vi "Draw Target Vr2.vi"(1 "Color":u32(colorbox)=16448250, 2 "Thickness":i32=3, 3 "Original Image":T1(plugin-control)) -> (0 "Image Out":T1(plugin-control))   [LabVIEW 2012]
uses:
  <resource>/objmgr/IMAQImage.rc
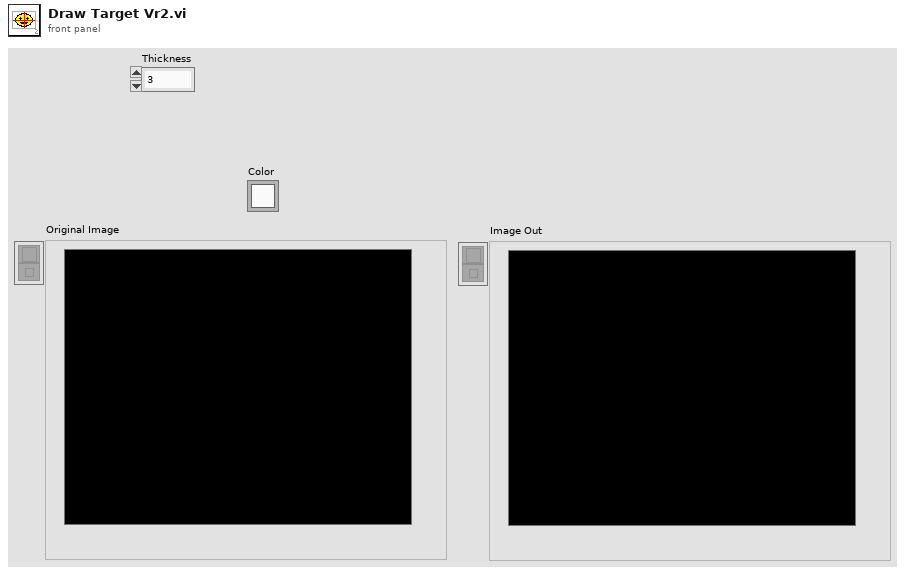
[diagram p1: front panel]
types:
  T1 = typedef "IMAQ Image.ctl" = refnum<image>
  T2 = cluster{"Left":i32, "Top":i32, "Right":i32, "Bottom":i32}
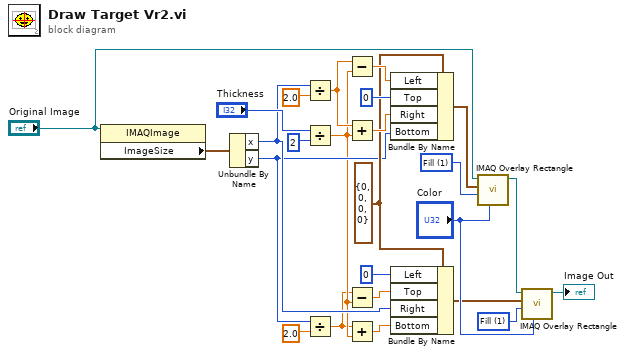
[diagram p0: block diagram]
diagram:
  w11 = u32 1 items=["Frame", "Fill", "Highlight"] ("Drawing Mode (Frame)")
  w16 = u32 1 items=["Frame", "Fill", "Highlight"] ("Drawing Mode (Frame)")
  w10 = T2 {"Left"=0, "Top"=0, "Right"=0, "Bottom"=0} ("Bounding Rectangle")
  n1 = property class="IMAQImage"(reference="Original Image") -> ("ImageSize"=w25:cluster{"x":i32, "y":i32})  [unwired: 1 in, 2 out]
  n2 = Unbundle By Name(w25) -> ("x"=w8:i32, "y"=w6:i32)
  n3 = Divide(x=w8, y=2.0) -> (x/y=w20:dbl)
  n4 = Divide(x="Thickness", y=2 ("x")) -> (x/y=w3:dbl)
  n5 = Divide(x=w6, y=2.0) -> (x/y=w2:dbl)
  n6 = Subtract(x=w20, y=w3) -> (x-y=w22:dbl)
  n7 = Add(x=w20, y=w3) -> (x+y=w19:dbl)
  n8 = Subtract(x=w2, y=w3) -> (x-y=w4:dbl)
  n9 = Add(x=w2, y=w3) -> (x+y=w5:dbl)
  n10 = Bundle By Name(cluster=w10, "Left"=w22, "Top"=0, "Right"=w19, "Bottom"=w6) -> (w18:T2)
  n11 = Bundle By Name(cluster=w10, "Left"=0, "Top"=w4, "Right"=w8, "Bottom"=w5) -> (w1:T2)
  n12 = call "IMAQ Overlay Rectangle"("Color"="Color", "Drawing Mode (Frame)"=w16, "Rectangle"=w18, "Image"="Original Image") -> ("Image Out"=w13:T1)  [unwired: 6 in, 1 out]
  n13 = call "IMAQ Overlay Rectangle"("Color"="Color", "Drawing Mode (Frame)"=w11, "Rectangle"=w1, "Image"=w13) -> ("Image Out"=→"Image Out":T1)  [unwired: 6 in, 1 out]
